vi "MAINP Get DBPath.vi"(8 "error in (no error)":errorcluster, 10 "Alias":string, 11 "Device Item Ref in":T1 format="%.0x") -> (0 "error out":errorcluster, 2 "Alias":string, 3 "Device Item Ref out":T1 format="%.0x", 5 "Path":string)   [LabVIEW 2018, in "CAN Gateway System Explorer.lvlib"]
uses:
  CAN Gateway System Explorer.lvlib
  <vilib>/NI Veristand/Custom Device API/Custom Device Item Ref.ctl
  <vilib>/NI Veristand/Custom Device API/Custom Device API.lvlib
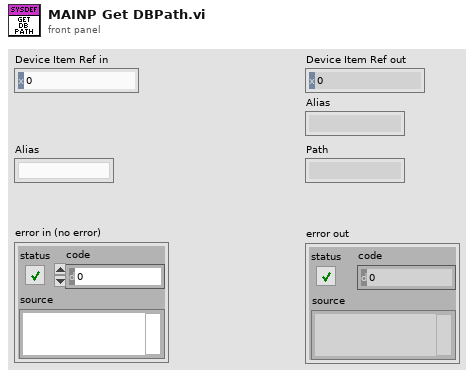
[diagram p1: front panel]
types:
  T1 = typedef "Custom Device API.lvlib/Custom Device Item Ref.ctl" = u64
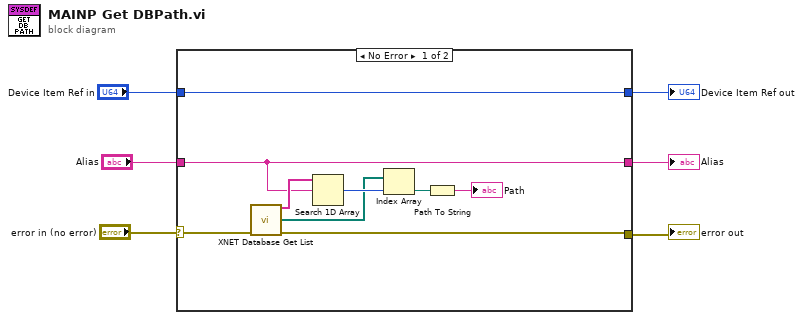
[diagram p0: block diagram]
diagram:
  n1 = case shown="No Error" "error in (no error)" {
    selector: "error in (no error)" -> [w15 w18]
    tunnel: "Device Item Ref in" -> [w10 w17]
    tunnel: [w10 w17] -> w4
    tunnel: [w11 w18] -> w3
    tunnel: "Alias" -> [w7 w16]
    tunnel: [w7 w16] -> w1
    frame No Error {
      n2 = call <vilib>:"XNET Database Get List.vi"("error in (no error)"=w15) -> ("array of alias"=w14:string[], "array of filepath"=w12:path[], "error out"=w11:errorcluster)  [unwired: 12 in]
      n3 = Search 1D Array(1D array=w14, element=w7) -> (index of element=w13:i32)  [unwired: 1 in]
      n4 = Index Array(array=w12, index=w13) -> (element=w9:path)
      n5 = Path To String(path=w9) -> (string=→"Path":string)
    }
    frame Error {
    }
  }
  "error out" <- w3
  "Device Item Ref out" <- w4
  "Alias" <- w1
